vi "mainPanel - Copie.vi"() -> ()   [LabVIEW 2024]
uses:
  <vilib>/Math Plots/3D Math Plots/3D Pie/3D Pie XCtrl/3D Pie.xctl
  <vilib>/Math Plots/3D Math Plots/3D Pie/3D Pie Datatype/Public/Plot Helper (Vector).vi
  <vilib>/Math Plots/3D Math Plots/3D Pie/3D Pie Datatype/3D Pie Datatype.lvclass
panel:
  in  "Tab Control":enum32{"A", "B", "B 2", "B 3"}(tab)
  in  "Path":path
  out "Image":T1(plugin-control)
  out "Nombre de véhicules:":dbl
  out "Nombre de \nvéhicules suspects:":dbl
  out "Localisation":string
  out "Date":string
  out "Nombre de véhicules Total":string
  out "Nombre véhicules Suspects":string
  out "Taux d'embouteillage":dbl(knob) scale=0.0..100.0
  out "Horaire":string[](array[string])
  out "Immatricule":string[](array[string])
  out "Dernière Alerte de suspection":string
  out "new picture 2":picture
  out "Nombre de véhicules Total":refnum<class "3D Plot Datatype.lvclass">[](xcontrol)
  out "String":string
  out "String 2":string
  in  "Quit":bool
  # "DIRECT"
  # "BILAN"
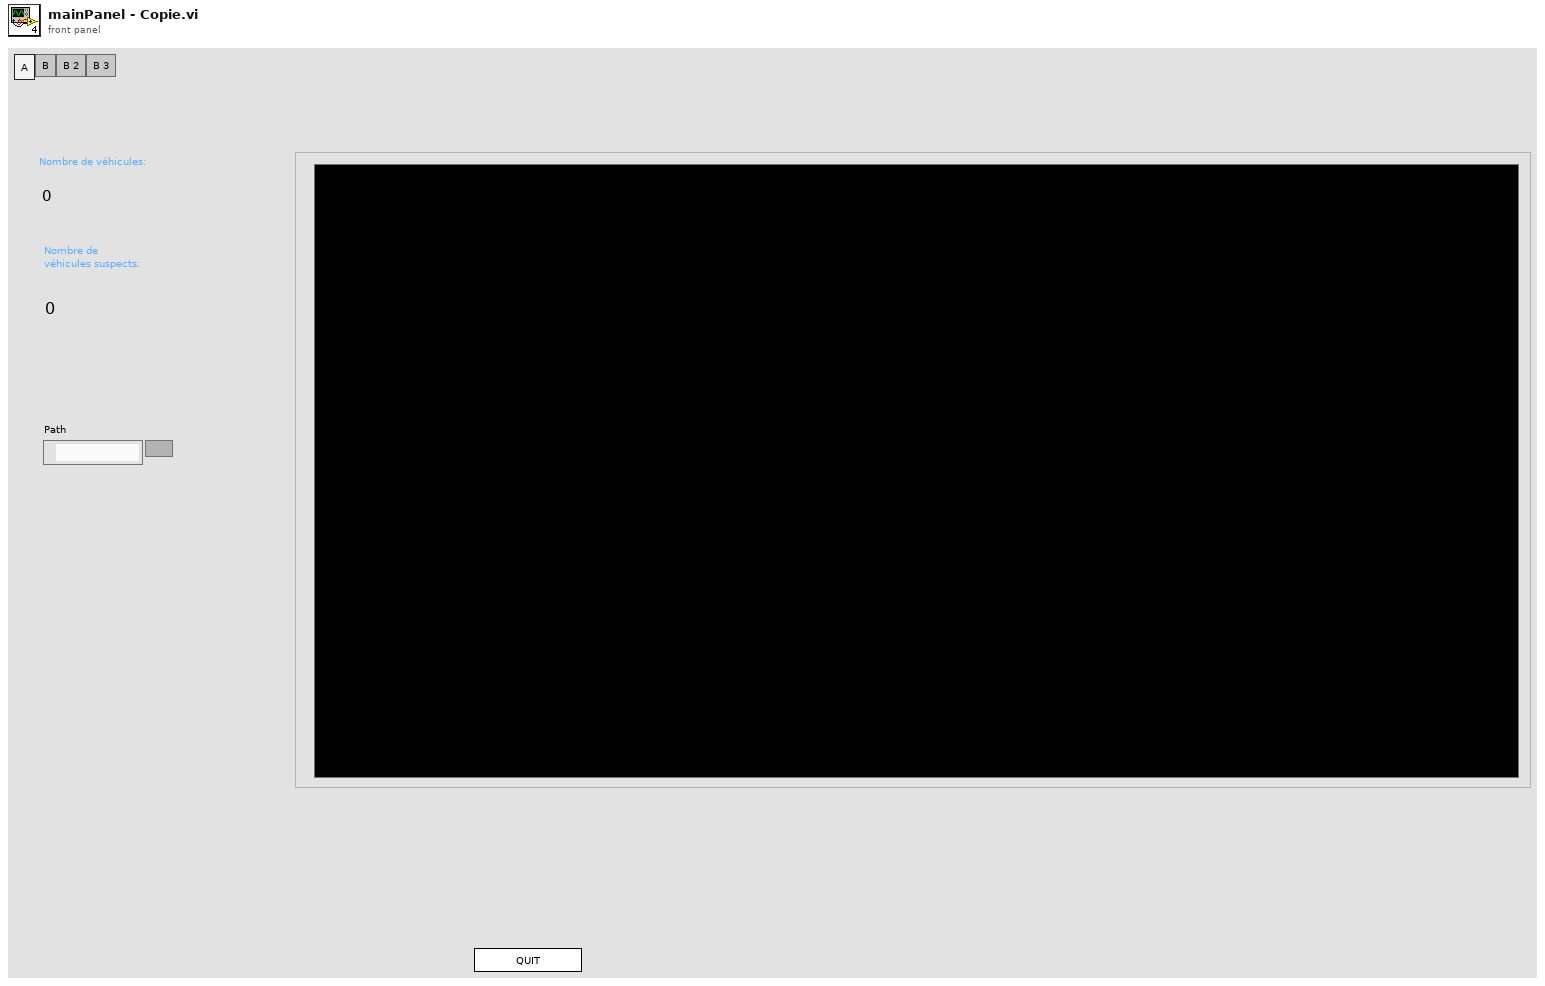
[diagram p1: front panel]
types:
  T1 = typedef "IMAQ Image.ctl" = refnum<image>
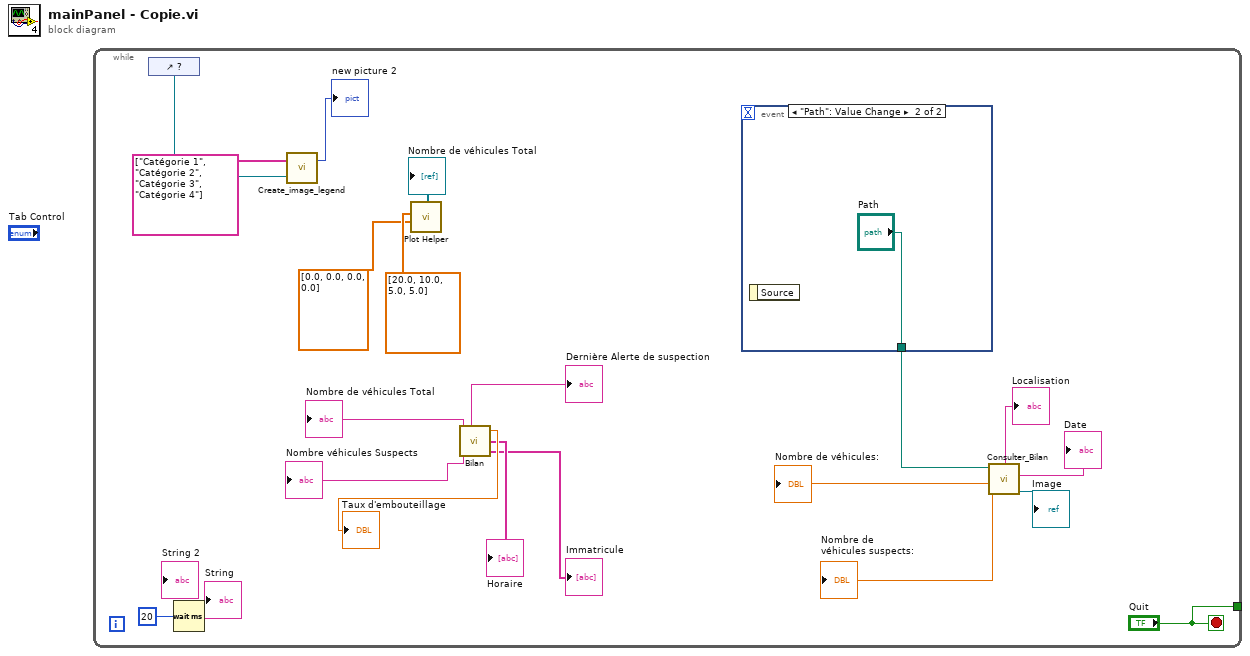
[diagram p0: block diagram]
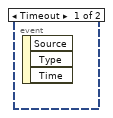
[diagram p2: hidden frame]
diagram:
  n1 = while {
    tunnel: ["Quit"] -> _
    stop <- "Quit" stop-if-true
    n2 = control-ref of="?"() -> (w8:refnum<vi>)
    n3 = Wait (ms)(milliseconds to wait=u32 20) -> ()  [unwired: 1 out]
    n4 = call "Create_image_legend.vi"("Nombre de véhicules Total 2"=w8, "Immatricule"=string[] ["Catégorie 1", "Catégorie 2", "Catégorie 3", "Catégorie 4"]) -> ("new picture"=→"new picture 2":picture)  [unwired: 1 in]
    n5 = call-poly <vilib>:"Plot Helper.vi"("offset vector"=dbl[] [0.0, 0.0, 0.0, 0.0], "x vector"=dbl[] [20.0, 10.0, 5.0, 5.0]) -> ("3D Plot lvclass Array out"=→"Nombre de véhicules Total":refnum<class "3D Plot Datatype.lvclass">[])  [unwired: 1 in, 8 out]
    n6 = call "Bilan.vi"() -> ("Nombre de véhicules Total"=→"Nombre de véhicules Total":string, "Nombre véhicules Suspects"=→"Nombre véhicules Suspects":string, "Dernière Alerte de suspection"=→"Dernière Alerte de suspection":string, "Taux d'embouteillage"=→"Taux d'embouteillage":dbl, "Horaire"=→"Horaire":string[], "Immatricule"=→"Immatricule":string[])  [unwired: 2 in]
    n7 = event shown="[1] \"Path\": Value Change" {
      selector: _ -> [_ _]
      dyn-events: _ -> [_ _]
      timeout: _ -> [_ _]
      tunnel: [_ "Path"] -> w1
      event Timeout {
        n8 = event-data() -> ()  [unwired: 1 in, 3 out]
      }
      event "Path": Value Change {
        n9 = event-data() -> ()  [unwired: 1 in, 1 out]
      }
    }
    n10 = call "Consulter_Bilan.vi"("File Path 2"=w1) -> ("Date"=→"Localisation":string, "Nombre de véhicules:"=→"Nombre de véhicules:":dbl, "Nombre de \nvéhicules suspects:"=→"Nombre de \nvéhicules suspects:":dbl, "Localisation"=→"Date":string, "Image"=→"Image":T1)  [unwired: 5 in]
  }
